vi "Write DAQmx Synthesizer Configuration.vi"(8 "error in (no error)":errorcluster, 10 "Configuration":T1={"Ranges"=[10.0], "Channel names"=[], "Output channels"="0:1", "File Path Control"=path "", "Offset"=1.0, "Scale"=0.5} {"Ranges" format="%#_6pV"}, 11 "DAQmx Synthesizer in":refnum<class "DAQmx Synthesizer.lvclass">) -> (0 "error out":errorcluster, 3 "DAQmx Synthesizer out":refnum<class "DAQmx Synthesizer.lvclass">)   [LabVIEW 2021, in "DAQmx Synthesizer.lvclass"]
uses:
  DAQmx Synthesizer.lvclass
  C:/GitHub/NHMFL_Core/Libraries/Instruments/Instrument Driver/Instrument Driver.lvclass
  DAQmx Synthesizer Configuration.ctl
  Instruments/Instrument Driver/Write User configuration.vi
  DAQmx Synthesizer.lvclass/DAQmx Synthesizer.ctl
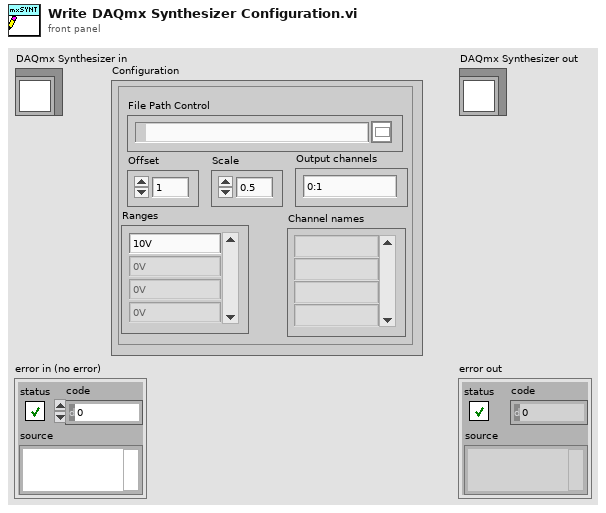
[diagram p1: front panel]
types:
  T1 = typedef "DAQmx Synthesizer Configuration.ctl" = cluster{"Ranges":dbl[], "Channel names":string[], "Output channels":string, "File Path Control":path, "Offset":dbl, "Scale":dbl}
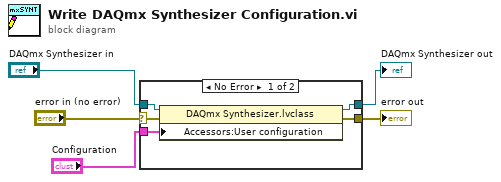
[diagram p0: block diagram]
diagram:
  n1 = case shown="No Error" "error in (no error)" {
    selector: "error in (no error)" -> [w10 w11]
    tunnel: [w9 w11] -> w4
    tunnel: [w7 w12] -> w2
    tunnel: "DAQmx Synthesizer in" -> [w8 w12]
    tunnel: "Configuration" -> [w6 _]
    frame No Error {
      n2 = property class="DAQmx Synthesizer.lvclass"(reference=w8, error in=w10, "Accessors:User configuration"=w6) -> (reference out=w7:refnum<class "DAQmx Synthesizer.lvclass">, error out=w9:errorcluster)
    }
    frame Error {
    }
  }
  "error out" <- w4
  "DAQmx Synthesizer out" <- w2
